vi "Dashboard Main.vi"() -> ()   [LabVIEW 2025]
panel:
  out "Camera Perf":string
  in  "Camera Settings":T1={"Frame Rate"=30, "Compression"=30, "Size"=1, "DB Camera Config"=FALSE} {"Frame Rate" scale=1.0..30.0; "Compression" scale=100.0..-1.0; "Size" items=["640x480", "320x240", "160x120"]}
  in  "TCP":refnum<k5>
  in  "Dashboard Tab":enum32{"Drive", "Basic", "Custom", "Variables"}(tab)
  in  "Select Auto":string(combo)="Select Autonomous ..."
  out "NT Connection":bool
  out "Mode":T2(ring)=enum."Auto Disabled"
  out "Robot IP":string
  out "DriverTest/TimeSinceCmd":dbl caption="Elapsed Time Since Cmd (Sec)" format="%21.3f"
  out "DriverTest/ElapsedSec":dbl caption="Elapsed Test Time (Sec)" format="%21.3f"
  out "DriverTest/Started":bool caption="Test Started"
  in  "DriverTest/Start":bool caption="Start Test"
  in  "DriverTest/Name":string caption="Drivers Name"
  in  "DriverTest/Stop":bool caption="Stop Test"
  out "Tree":string(tree)
  out "Camera Image":T3(plugin-control)
  in  "Camera Name":string(combo)="No Camera Selection"
  # "HW"
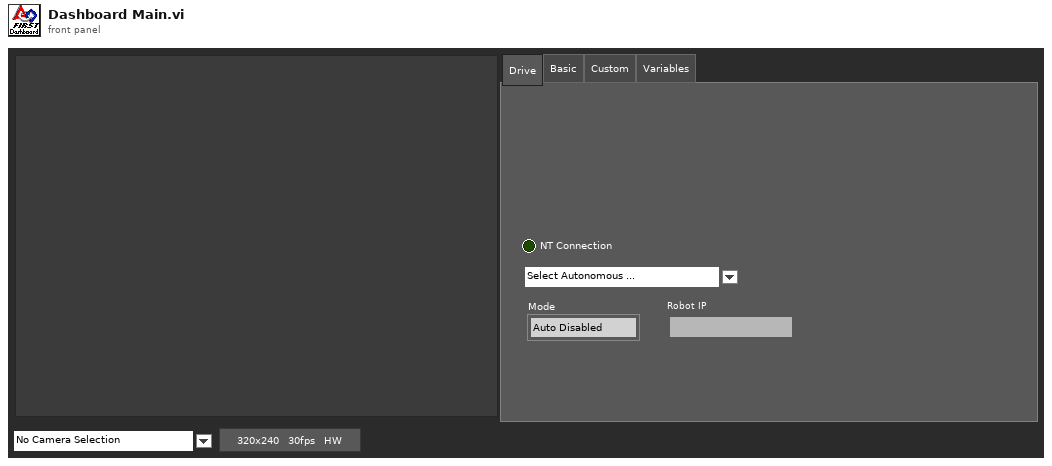
[diagram p1: front panel]
types:
  T1 = cluster{"Frame Rate":i32, "Compression":i32, "Size":u16, "DB Camera Config":bool}
  T2 = enum8{"Tele-Op Disabled", "Tele-Op Enabled", "Auto Disabled", "Auto Enabled", "Test Disabled", "Test Enabled", "Disconnected", "No Code", "E-Stop"}
  T3 = typedef "IMAQ Image.ctl" = refnum<image>
  T4 = cluster{"Save Path":path, "Interval (s)":dbl, "Keep":i32}
  T5 = typedef "Image Type" = u32
  T6 = cluster{"Shift":bool, "Ctrl":bool, "Alt":bool, "Cmd":bool, "Opt":bool}
  T7 = cluster{"Error Strings":string, "Disable Counts":cluster{u16, u16}, "Rail Faults":cluster{u16, u16, u16}, "Robot IP":string, "DB Mode":u8, "Event Info":cluster{"Name":string, "Type":u8, "Number":u16, "Replay":u8}}
  T8 = cluster{"Storage":cluster{"Disk Free":u64, "RAM Block":u32, "RAM free":u32}, "CPU Utilization":cluster{"CPU % ISR":sgl, "CPU % Time Crit":sgl, "CPU % Timed Str":sgl, "CPU % High":sgl, "CPU % Above":sgl, "CPU % Normal":sgl, "CPU % Low":sgl}, "CAN":cluster{"% Bus Utilization":sgl, "Bus Off Cnt":u32, "TX_FIFO Full Cnt":u32, "Receive Error Cnt":u8, "Transmit Error Cnt":u8}, "HID":cluster{"HID Outputs":u32, "Rumble Low":u16, "Rumble High":u16}[]}
  T9 = cluster{"Status bits":cluster{"Test Mode":bool, "Autonomous":bool, "Enabled":bool, "Code Start":bool, "Brownout":bool, "Reserved 2":bool, "Reserved 3":bool, "E-Stop":bool}, "Code Trace":cluster{"Disabled":bool, "TeleOp":bool, "Auto":bool, "Test":bool}, "Controller Type":enum16{"unknown", "cRIO", "roboRio"}, "Code?":enum16{"unknown", "noCode", "code"}, "Battery V":dbl}
  T10 = cluster{"Control Bits":cluster{"TestMode":bool, "Autonomous":bool, "Enabled":bool, "FMS Present":bool, bool, bool, bool, "E-Stop":bool}, "Team Station ":u8, "Countdown":sgl, "Joystick Values":cluster{"Axes":dbl[], "Buttons":bool[], "POVs":i16[]}[]}
  T11 = cluster{"Camera Name":string, "Camera File Name":string, "Saved DB Images Info":cluster{"Save Path":path, "Interval (s)":dbl, "Keep":i32}}
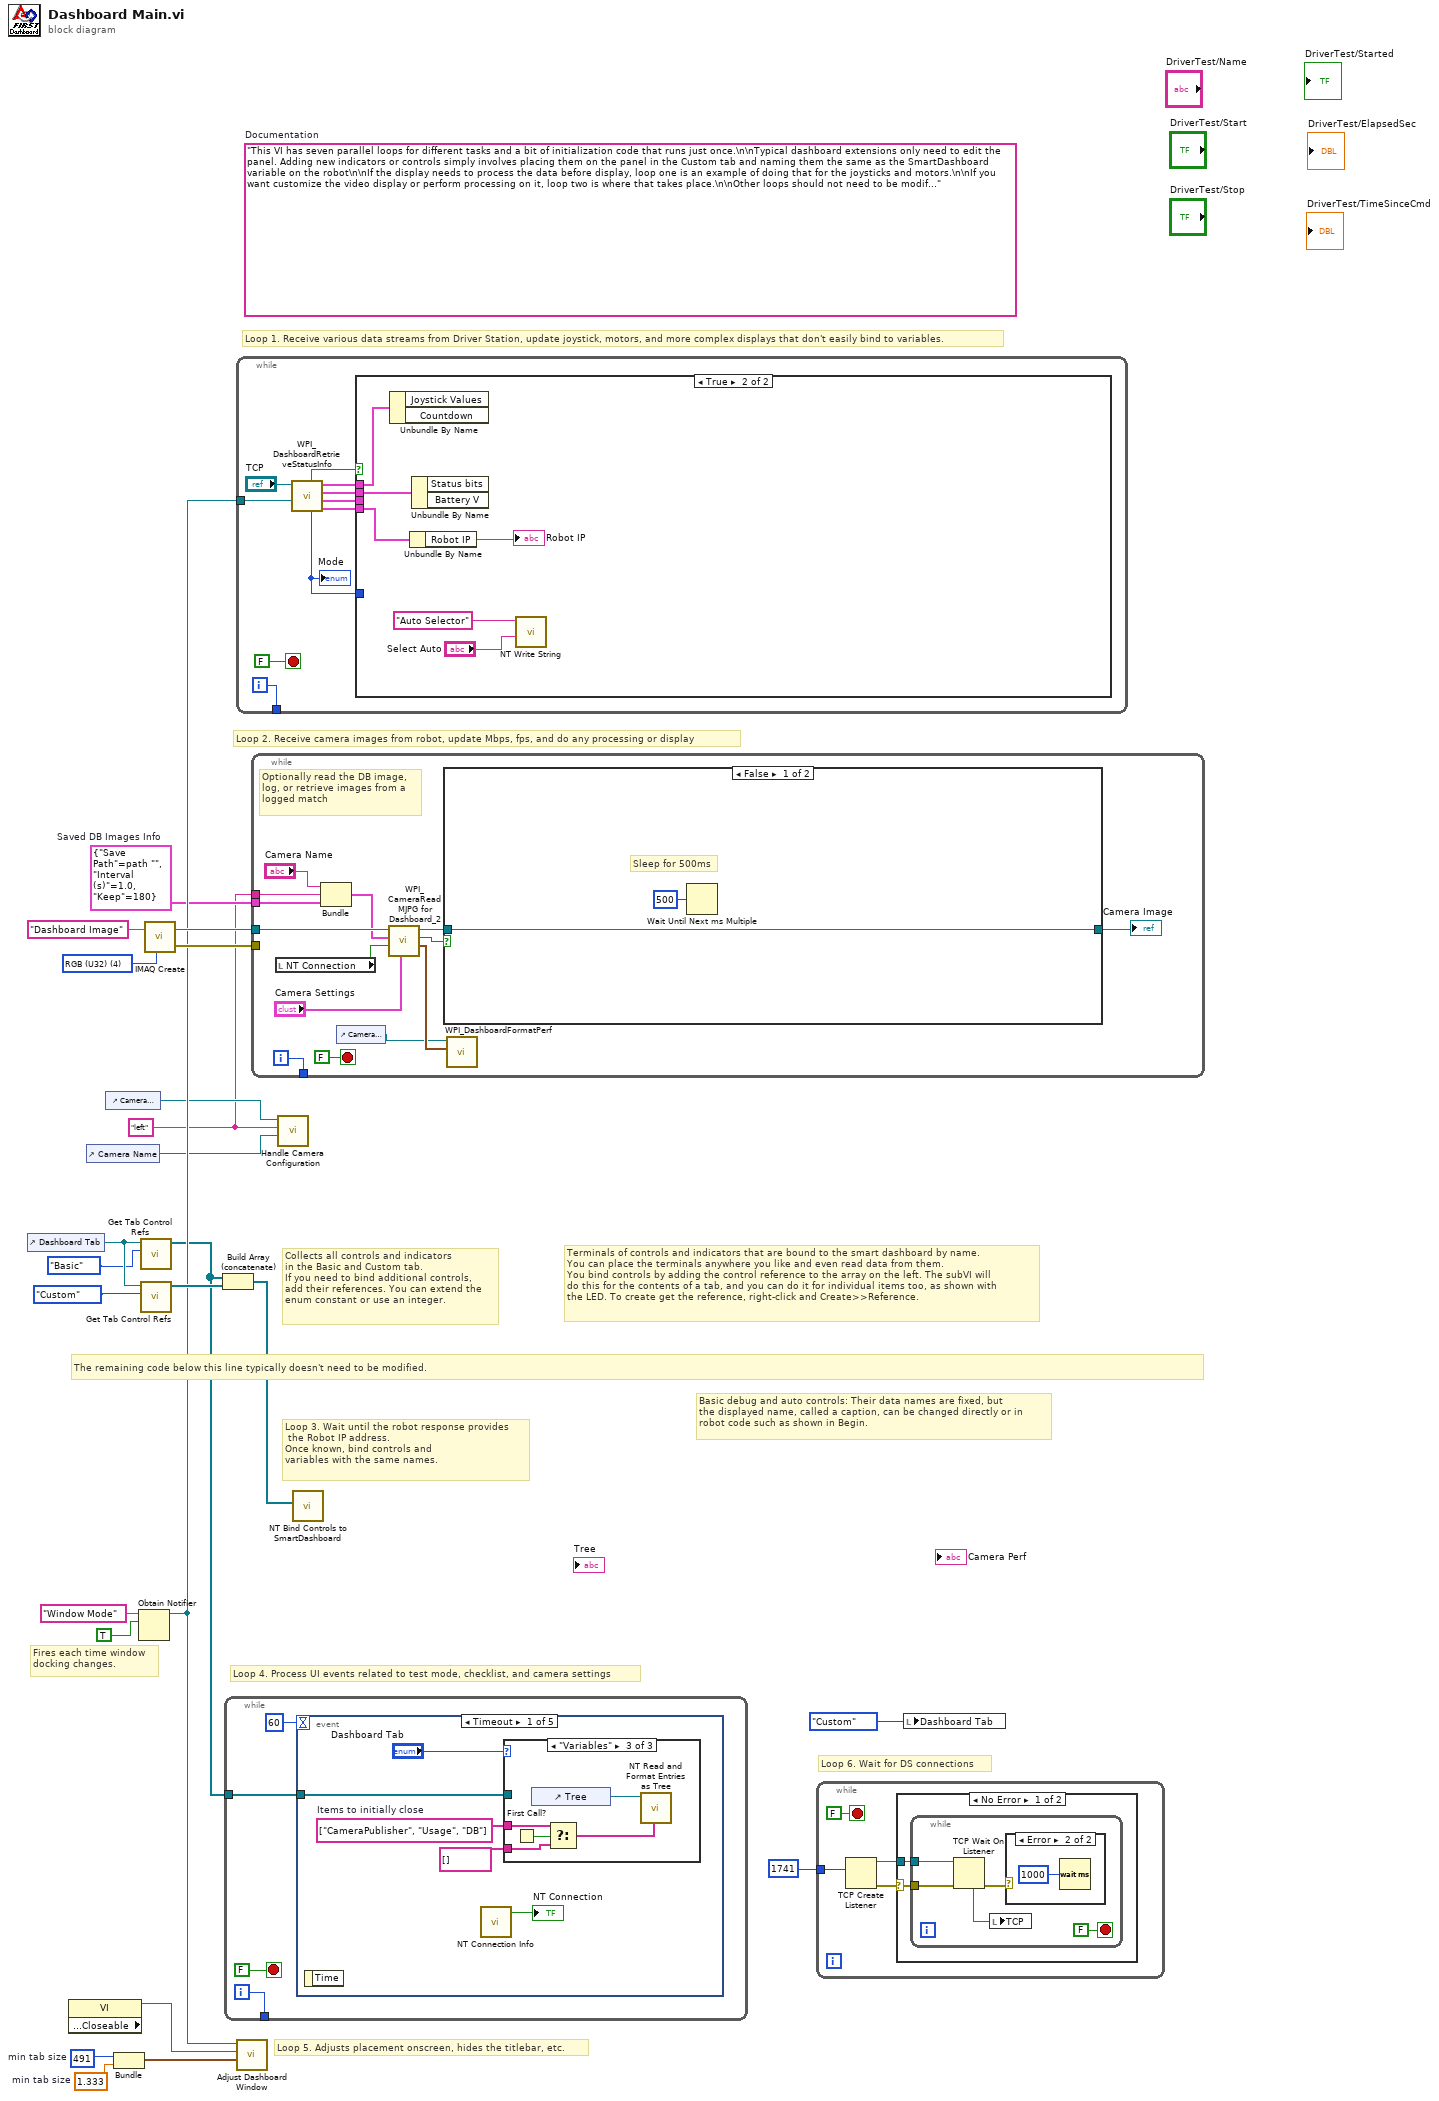
[diagram p0: block diagram]
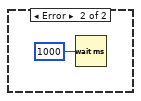
[diagram p3: hidden frame]
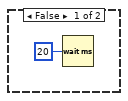
[diagram p4: hidden frame]
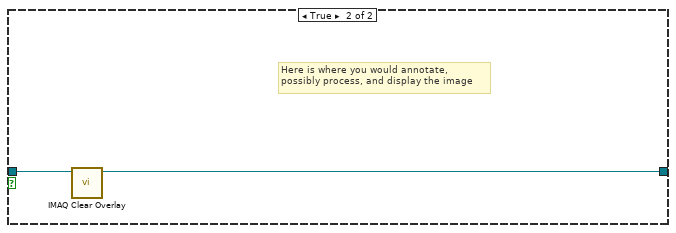
[diagram p5: hidden frame]
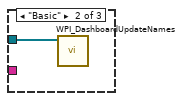
[diagram p7: hidden frame]
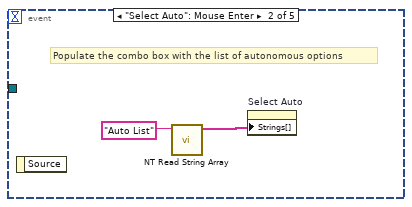
[diagram p8: hidden frame]
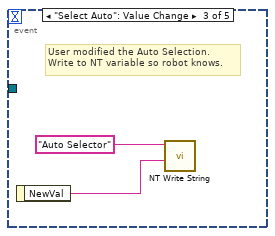
[diagram p9: hidden frame]
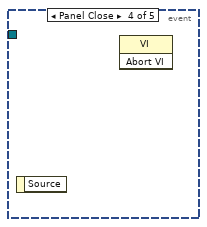
[diagram p10: hidden frame]
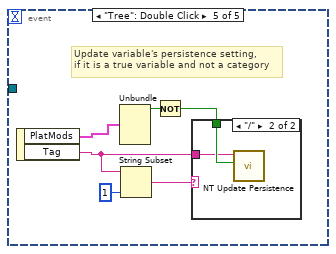
[diagram p11: hidden frame]
diagram:
  w2 = "left" ("Camera File Name")
  w3 = T4 {"Save Path"=path "", "Interval (s)"=1.0, "Keep"=180}  # Saved DB Images Info
  w13 = 491  # min tab size
  w12 = 1.333  # min tab size
  (unwired) "This VI has seven parallel loops for different tasks and a bit of initialization code that runs just once.\n\nTypical dashboard extensions only need to edit the panel. Adding new indicators or controls simply involves placing them on the panel in the Custom tab and naming them the same as the SmartDashboard variable on the robot\n\nIf the display needs to process the data before display, loop one is an example of doing that for the joysticks and motors.\n\nIf you want customize the video display or perform processing on it, loop two is where that takes place.\n\nOther loops should not need to be modified. They are pretty standard, and document the task they perform."  # Documentation
  w23 = T5 4 items=["Grayscale (U8)", "Grayscale (I16)", "Grayscale (SGL)", "Complex (CSG)", "RGB (U32)", "HSL (U32)", "RGB (U64)"] ("Image Type")
  # "Loop 6. Wait for DS connections"
  # "Basic debug and auto controls: Their data names are fixed, but\nthe displayed name, called a caption, can be changed directly or in\nrobot code such as shown in Begin."
  # "Fires each time window\ndocking changes."
  # "Collects all controls and indicators\nin the Basic and Custom tab.\nIf you need to bind additional controls,\nadd their references. You can extend the\nenum constant or use an integer."
  # "The remaining code below this line typically doesn't need to be modified."
  # "Loop 4. Process UI events related to test mode, checklist, and camera settings"
  # "Terminals of controls and indicators that are bound to the smart dashboard by name.\nYou can place the terminals anywhere you like and even read data from them.\nYou bind controls by adding the control reference to the array on the left. The subVI will\ndo this for the contents of a tab, and you can do it for individual items too, as shown with\nthe LED. To create get the reference, right-click and Create>>Reference."
  # "Loop 3. Wait until the robot response provides\n the Robot IP address.\nOnce known, bind controls and\nvariables with the same names."
  # "Loop 5. Adjusts placement onscreen, hides the titlebar, etc."
  # "Loop 1. Receive various data streams from Driver Station, update joystick, motors, and more complex displays that don't easily bind to variables."
  # "Loop 2. Receive camera images from robot, update Mbps, fps, and do any processing or display"
  n1 = control-ref of="Dashboard Tab"() -> (w16:refnum<vi>)
  n2 = property class="VI" props=["Front Panel.Closeable"]() -> (reference out=w17:refnum<vi>)  [unwired: 2 in, 2 out]
  n3 = control-ref of="Camera Name"() -> (w7:refnum<vi>)
  n4 = control-ref of="Camera Settings"() -> (w8:refnum<vi>)
  n5 = Bundle("min tab size"=w13, "min tab size"=w12) -> (w11:cluster{"min tab size":i32, "min tab size":dbl})  [unwired: 1 in]
  n6 = Obtain Notifier(name (unnamed)="Window Mode", notification data type=TRUE) -> (notifier out=w10:refnum<notifier>)  [unwired: 2 in, 2 out]
  n7 = call <vilib>:"Get Tab Control Refs.vi"("Page Index"=enum32{"Drive", "Basic", "Custom", "Variables"}."Basic" ("Dashboard Tab"), "TabControl in"=w16) -> ("ControlsOnPage"=w6:refnum<vi>[])  [unwired: 9 in]
  n8 = call <vilib>:"Get Tab Control Refs.vi"("Page Index"=enum32{"Drive", "Basic", "Custom", "Variables"}."Custom" ("Dashboard Tab"), "TabControl in"=w16) -> ("ControlsOnPage"=w15:refnum<vi>[])  [unwired: 9 in]
  n9 = call "IMAQ Create"("Image Name"="Dashboard Image", "Image Type"=w23) -> ("New Image"=w21:T3, "error out"=w20:errorcluster)  [unwired: 2 in, 1 out]
  n10 = Build Array (concatenate)(w6, w15) -> (w14:refnum<vi>[])
  n11 = while {
    tunnel: [w25] -> _
    tunnel: w6 -> [w24]
    i -> [w25]
    stop <- FALSE stop-if-true
    n12 = event shown="[0] Timeout" {
      selector: _ -> [_ _ _ _ _]
      dyn-events: _ -> [_ _ _ _ _]
      timeout: u32 60 ("milliseconds to wait") -> [_ _ _ _ _]
      tunnel: w24 -> [w31 _ _ _ _]
      event Timeout {
        w30 = string[] ["CameraPublisher", "Usage", "DB"]  # Items to initially close
        n13 = event-data() -> ()  [unwired: 1 in, 1 out]
        n14 = call <vilib>:"NT Connection Info.vi"() -> ("Connected"=→"NT Connection":bool)  [unwired: 11 in]
        n15 = case shown="\"Variables\"" "Dashboard Tab" {
          tunnel: w31 -> [_ w33 _]
          tunnel: w30 -> [_ _ w36]
          tunnel: string[] [] -> [_ _ w35]
          frame "Custom", Default {
          }
          frame "Basic" {
            n16 = call <vilib>:"WPI_DashboardUpdateNames.vi"("Controls on Tab"=w33) -> ()  [unwired: 11 in]
          }
          frame "Variables" {
            n17 = First Call?() -> (First Call?: T/F=w37:bool)
            n18 = control-ref of="Tree"() -> (w38:refnum<vi>)
            n19 = Select(t=w36, s=w37, f=w35) -> (s? t:f=w34:string[])
            n20 = call <vilib>:"NT Read and Format Entries as Tree.vi"("Tags to  Close"=w34, "Tree Refnum"=w38) -> ()  [unwired: 8 in, 2 out]
          }
        }
      }
      event "Select Auto": Mouse Enter {
        # "Populate the combo box with the list of autonomous options"
        n21 = event-data() -> ()  [unwired: 1 in, 1 out]
        n22 = call <vilib>:"NT Read String Array.vi"("name"="Auto List" ("Name")) -> ("value"=w39:string[])  [unwired: 8 in, 2 out]
        n23 = property on="Select Auto" class="CmbBox"("Strings[]"=w39) -> ()  [unwired: 2 in, 2 out]
      }
      event "Select Auto": Value Change {
        # "User modified the Auto Selection.\nWrite to NT variable so robot knows."
        n24 = event-data() -> ("NewVal"=w41:string)  [unwired: 1 in]
        n25 = call <vilib>:"NT Write String.vi"("value"=w41, "name"="Auto Selector" ("Name")) -> ()  [unwired: 9 in, 1 out]
      }
      event Panel Close {
        n26 = event-data() -> ()  [unwired: 1 in, 1 out]
        n27 = invoke class="VI" method="Abort VI"() -> ()  [unwired: 3 in, 3 out]
      }
      event "Tree": Double Click {
        # "Update variable's persistence setting,\nif it is a true variable and not a category"
        n28 = event-data() -> ("PlatMods"=w44:T6, "Tag"=w43:string)  [unwired: 1 in]
        n29 = Unbundle(w44) -> ("Shift"=w48:bool)  [unwired: 4 out]
        n30 = String Subset(string=w43, length (rest)=1 ("length (rest)")) -> (substring=w45:string)  [unwired: 1 in]
        n31 = Not(x=w48) -> (.not. x?=w47:bool)
        n32 = case shown="\"/\"" w45 {
          tunnel: w47 -> [_ w50]
          tunnel: w43 -> [_ w49]
          frame Default {
          }
          frame "/" {
            n33 = call <vilib>:"NT Update Persistence.vi"("Persistence"=w50, "Name"=w49) -> ()  [unwired: 9 in, 1 out]
          }
        }
      }
    }
  }
  n34 = while {
    tunnel: [w59] -> _
    tunnel: w10 -> [w51]
    i -> [w59]
    stop <- FALSE stop-if-true
    n35 = call <vilib>:"WPI_DashboardRetrieveStatusInfo.vi"("Window Mode Notifier"=w51, "TCP Cnx"="TCP") -> ("Power and Errors"=w54:T7, "Robot Metrics"=w57:T8, "Status Info"=w58:T9, "Control Info"=w55:T10, "Robot Mode"=w53:T2, "Process?"=w56:bool)  [unwired: 4 in]
    "Mode" <- w53
    n36 = case shown="True" w56 {
      tunnel: w58 -> [_ w67]
      tunnel: w57 -> [_ _]
      tunnel: w55 -> [_ w66]
      tunnel: w54 -> [_ w65]
      tunnel: w53 -> [_ _]
      frame False {
        n37 = Wait (ms)(milliseconds to wait=u32 20) -> ()  [unwired: 1 out]
      }
      frame True {
        n38 = Unbundle By Name(w66) -> ()  [unwired: 2 out]
        n39 = Unbundle By Name(w65) -> ("Robot IP"=→"Robot IP":string)
        n40 = Unbundle By Name(w67) -> ()  [unwired: 2 out]
        n41 = call <vilib>:"NT Write String.vi"("value"="Select Auto", "name"="Auto Selector" ("Name")) -> ()  [unwired: 9 in, 1 out]
      }
    }
  }
  n42 = call "Adjust Dashboard Window.vi"("Size Constraints"=w11, "VI"=w17, "WIn Mode"=w10) -> ()  [unwired: 9 in]
  n43 = while {
    tunnel: w21 -> [w79]
    tunnel: w20 -> [_]
    tunnel: [w80] -> _
    tunnel: w3 -> [w73]
    tunnel: w2 -> [w70]
    i -> [w80]
    stop <- FALSE stop-if-true
    # "Optionally read the DB image,\nlog, or retrieve images from a\nlogged match"
    n44 = local read "NT Connection"() -> (w74:bool)
    n45 = Bundle("Camera Name"="Camera Name", "Camera File Name"=w70, "Saved DB Images Info"=w73) -> (w72:T11)  [unwired: 1 in]
    n46 = control-ref of="Camera Perf"() -> (w68:refnum<vi>)
    n47 = call <vilib>:"WPI_CameraRead MJPG for Dashboard_2.vi"("Camera Settings"="Camera Settings", "NT Connection"=w74, "Capture Info"=w72, "Image in"=w79) -> ("perf info"=w69:cluster{"Bandwidth (Mbps)":dbl, "fps":dbl}, "Active"=w77:bool, "Image\\ out"=w78:T3)  [unwired: 5 in]
    n48 = case shown="False" w77 {
      tunnel: w78 -> [w82 w85]
      tunnel: [w82 w84] -> w75
      frame False {
        # "Sleep for 500ms"
        n49 = Wait Until Next ms Multiple(millisecond multiple=u32 500) -> ()  [unwired: 1 out]
      }
      frame True {
        # "Here is where you would annotate,\npossibly process, and display the image"
        n50 = call "IMAQ Clear Overlay"("Image"=w85) -> ("Image Out"=w84:T3)  [unwired: 2 in, 8 out]
      }
    }
    "Camera Image" <- w75
    n51 = call <vilib>:"WPI_DashboardFormatPerf.vi"("Performance"=w69, "String in"=w68) -> ()  [unwired: 10 in]
  }
  n52 = call "Handle Camera Configuration.vi"("CameraNameRef"=w7, "Display Name"=w2, "ClusterRef"=w8) -> ()  [unwired: 9 in]
  n53 = call <vilib>:"NT Bind Controls to SmartDashboard.vi"("Bound Control Refs"=w14) -> ()  [unwired: 11 in]
  n54 = while {
    tunnel: u16 1741 ("timeout ms (25000)") -> [w87]
    stop <- FALSE stop-if-true
    n55 = TCP Create Listener(10:w87) -> (0:w86:errorcluster, 3:w88:refnum<k5>)  [unwired: 4 in, 1 out]
    n56 = case shown="No Error" w86 {
      selector: w86 -> [w90 _]
      tunnel: w88 -> [w91 _]
      frame No Error {
        n57 = while {
          tunnel: w91 -> [w94]
          tunnel: w90 -> [w93]
          stop <- FALSE stop-if-true
          n58 = TCP Wait On Listener(8:w93, 11:w94) -> (0:w95:errorcluster, 4:w96:refnum<k5>)  [unwired: 2 in, 3 out]
          n59 = local write "TCP"(w96) -> ()
          n60 = case shown="Error" w95 {
            frame No Error {
            }
            frame Error {
              n61 = Wait (ms)(milliseconds to wait=u32 1000) -> ()  [unwired: 1 out]
            }
          }
        }
      }
      frame Error {
        n62 = Wait (ms)(milliseconds to wait=u32 1000) -> ()  [unwired: 1 out]
      }
    }
  }
  n63 = local write "Dashboard Tab"(enum32{"Drive", "Basic", "Custom", "Variables"}."Custom" ("Dashboard Tab")) -> ()
